vi "Day 21-Calculate Move and Score using Buffer.vi"(6 "Game Board Buffer":refnum<queue>[](array[refnum]), 7 "Player Turn":T1=enum."Player 2", 8 "Dice Roll Sum":u64) -> (1 "Points Earned":u64)   [LabVIEW 2021]
uses:
  Day 21-Player Turn.ctl
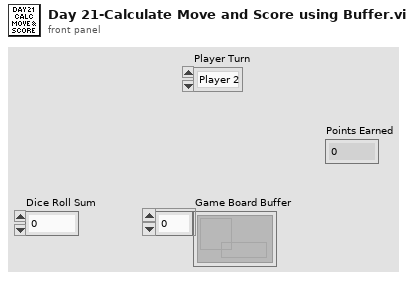
[diagram p1: front panel]
types:
  T1 = typedef "Day 21-Player Turn.ctl" = enum16{"Player 1", "Player 2"}
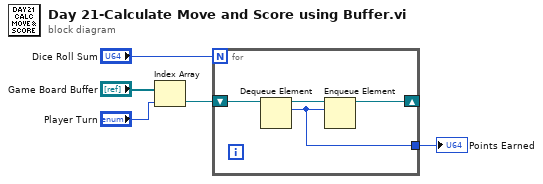
[diagram p0: block diagram]
diagram:
  n1 = Index Array(array="Game Board Buffer", index="Player Turn") -> (element=w4:refnum<queue>)
  n2 = for {
    N: "Dice Roll Sum" -> [_]
    shift-right: [w7] -> _
    shift-left: w4 -> [w9]
    tunnel: [w6] -> w1
    n3 = Dequeue Element(queue=w9) -> (queue out=w8:refnum<queue>, element=w6:u64)  [unwired: 2 in, 2 out]
    n4 = Enqueue Element(queue=w8, element=w6) -> (queue out=w7:refnum<queue>)  [unwired: 2 in, 2 out]
  }
  "Points Earned" <- w1
